vi "Scrape Module Configuration.vi"(8 "error in (no error)":errorcluster, 11 "SLSC Device":refnum<k21>) -> (0 "error out":errorcluster, 1 "switches json":string, 2 "topologies":string[](array[string]), 3 "product name":string, 4 "slot number":u32)   [LabVIEW 2017]
uses:
  <vilib>/SLSC/Initialize Session with Devices.vi
  <vilib>/SLSC/Close Session.vi
  <vilib>/SLSC_Switch/Get Topologies (Simulate).vi
  <resource>/objmgr/slsc.rc
  <vilib>/SLSC/SLSC.lvlib
  <vilib>/SLSC_Switch/SLSC Switch.lvlib
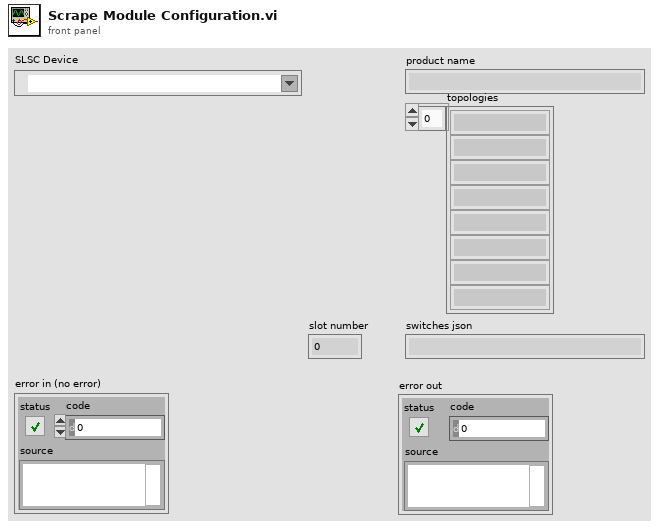
[diagram p1: front panel]
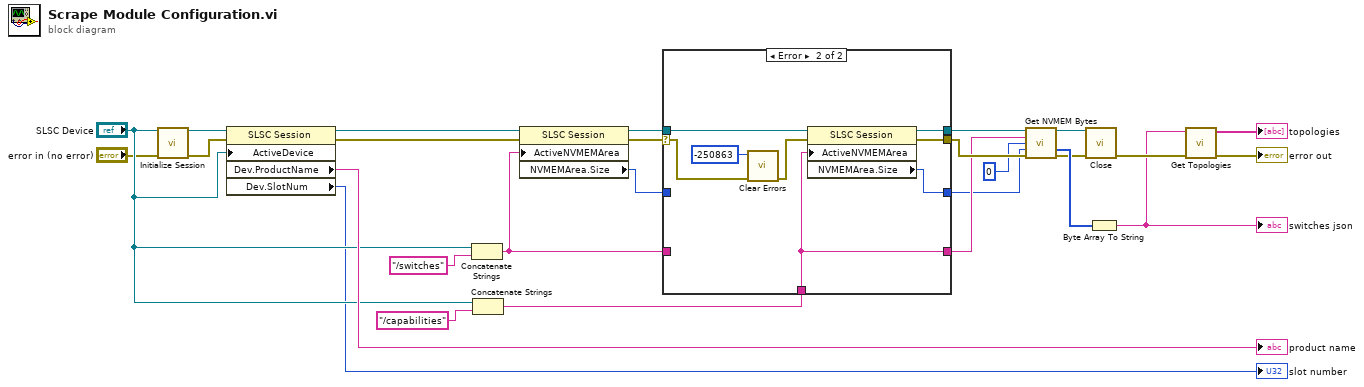
[diagram p0: block diagram]
diagram:
  n1 = call-poly <vilib>:"Initialize Session.vi"("devices"="SLSC Device", "error in (no error)"="error in (no error)") -> ("session out"=w27:refnum<k21>, "error out"=w26:errorcluster)  [unwired: 12 in]
  n2 = property class="SLSC Session"(reference=w27, error in=w26, "ActiveDevice"="SLSC Device") -> (reference out=w24:refnum<k21>, error out=w21:errorcluster, "Dev.ProductName"=→"product name":string, "Dev.SlotNum"=→"slot number":u32)
  n3 = Concatenate Strings("SLSC Device", "/switches" ("string")) -> (w15:string)
  n4 = Concatenate Strings("SLSC Device", "/capabilities" ("string")) -> (w17:string)
  n5 = property class="SLSC Session"(reference=w24, error in=w21, "ActiveNVMEMArea"=w15) -> (reference out=w18:refnum<k21>, error out=w22:errorcluster, "NVMEMArea.Size"=w16:u32)
  n6 = case shown="Error" w22 {
    selector: w22 -> [w28 w34]
    tunnel: w18 -> [w29 w39]
    tunnel: w17 -> [_ w37]
    tunnel: w16 -> [w30 _]
    tunnel: [w30 w38] -> w10
    tunnel: w15 -> [w31 _]
    tunnel: [w31 w37] -> w12
    tunnel: [w29 w36] -> w14
    tunnel: [w28 w35] -> w13
    frame No Error {
    }
    frame Error {
      n7 = call <vilib>:"Clear Errors.vi"("error in (no error)"=w34, "specific error code to clear (0: all)"=-250863) -> ("error out"=w33:errorcluster)  [unwired: 4 in, 1 out]
      n8 = property class="SLSC Session"(reference=w39, error in=w33, "ActiveNVMEMArea"=w37) -> (reference out=w36:refnum<k21>, error out=w35:errorcluster, "NVMEMArea.Size"=w38:u32)
    }
  }
  n9 = call <vilib>:"Get NVMEM Bytes.vi"("session in"=w14, "NVMEM area"=w12, "data address"=u32 0, "data size"=w10, "error in (no error)"=w13) -> ("session out"=w8:refnum<k21>, "data out"=w9:u8[], "error out"=w7:errorcluster)  [unwired: 6 in, 2 out]
  n10 = call-poly <vilib>:"Close.vi"("session in"=w8, "error in (no error)"=w7) -> ("error out"=w6:errorcluster)  [unwired: 13 in]
  n11 = Byte Array To String(unsigned byte array=w9) -> (string=w5:string)
  "switches json" <- w5
  n12 = call-poly <vilib>:"Get Topologies.vi"("error in (no error)"=w6, "switches json"=w5) -> ("error out"=→"error out":errorcluster, "topologies"=→"topologies":string[])  [unwired: 8 in]
